vi "MOCKBEAR_Pull_Sample.vi"(0 "MOCKBEAR in":refnum<class "MOCKBEAR.lvclass">, 1 "FEA Model":refnum<class "FEA_Model.lvclass">, 5 "error in (no error)":errorcluster) -> (12 "Frequency True":dbl, 14 "Accelerometer sample":dbl[](array[numeric]), 15 "Last pin pos node":i32, 16 "Sample Time":u32, 17 "Last pin pos meter":dbl, 18 "looping":bool, 19 "error out":errorcluster)   [LabVIEW 2021, in "MOCKBEAR.lvclass"]
uses:
  MOCKBEAR.lvclass
  FEA_Model/FEA_Model.lvclass
  MOCKBEAR.lvclass/MOCKBEAR.ctl
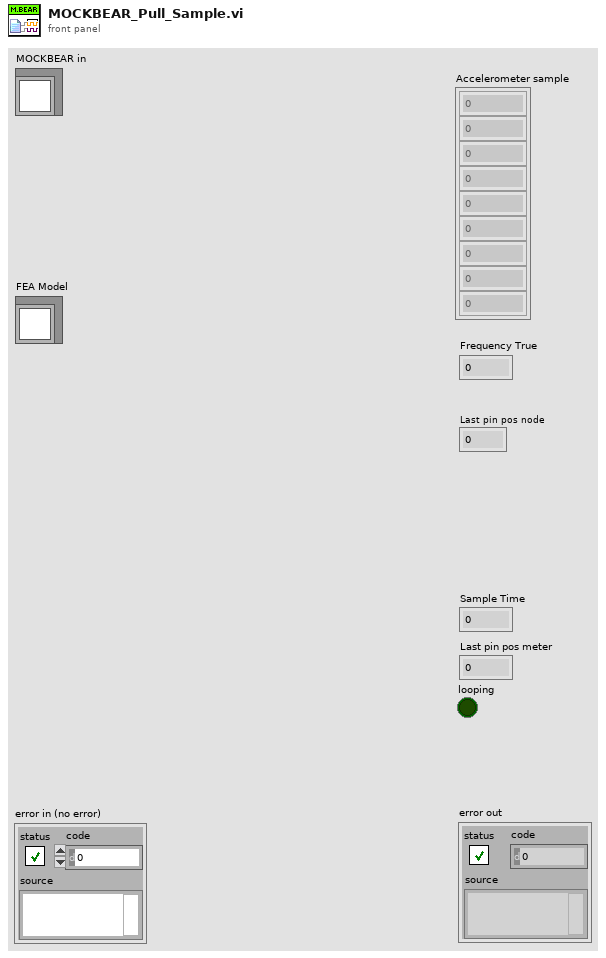
[diagram p1: front panel]
types:
  T1 = enum16{"Scalar Particle to Meter", "Scalar Node to Meter", "Scalar Meter to Particle", "Scalar Meter to Node", "Array Particle to Meter", "Array Node to Meter", "Array Meter to Particle", "Array Meter to Node"}
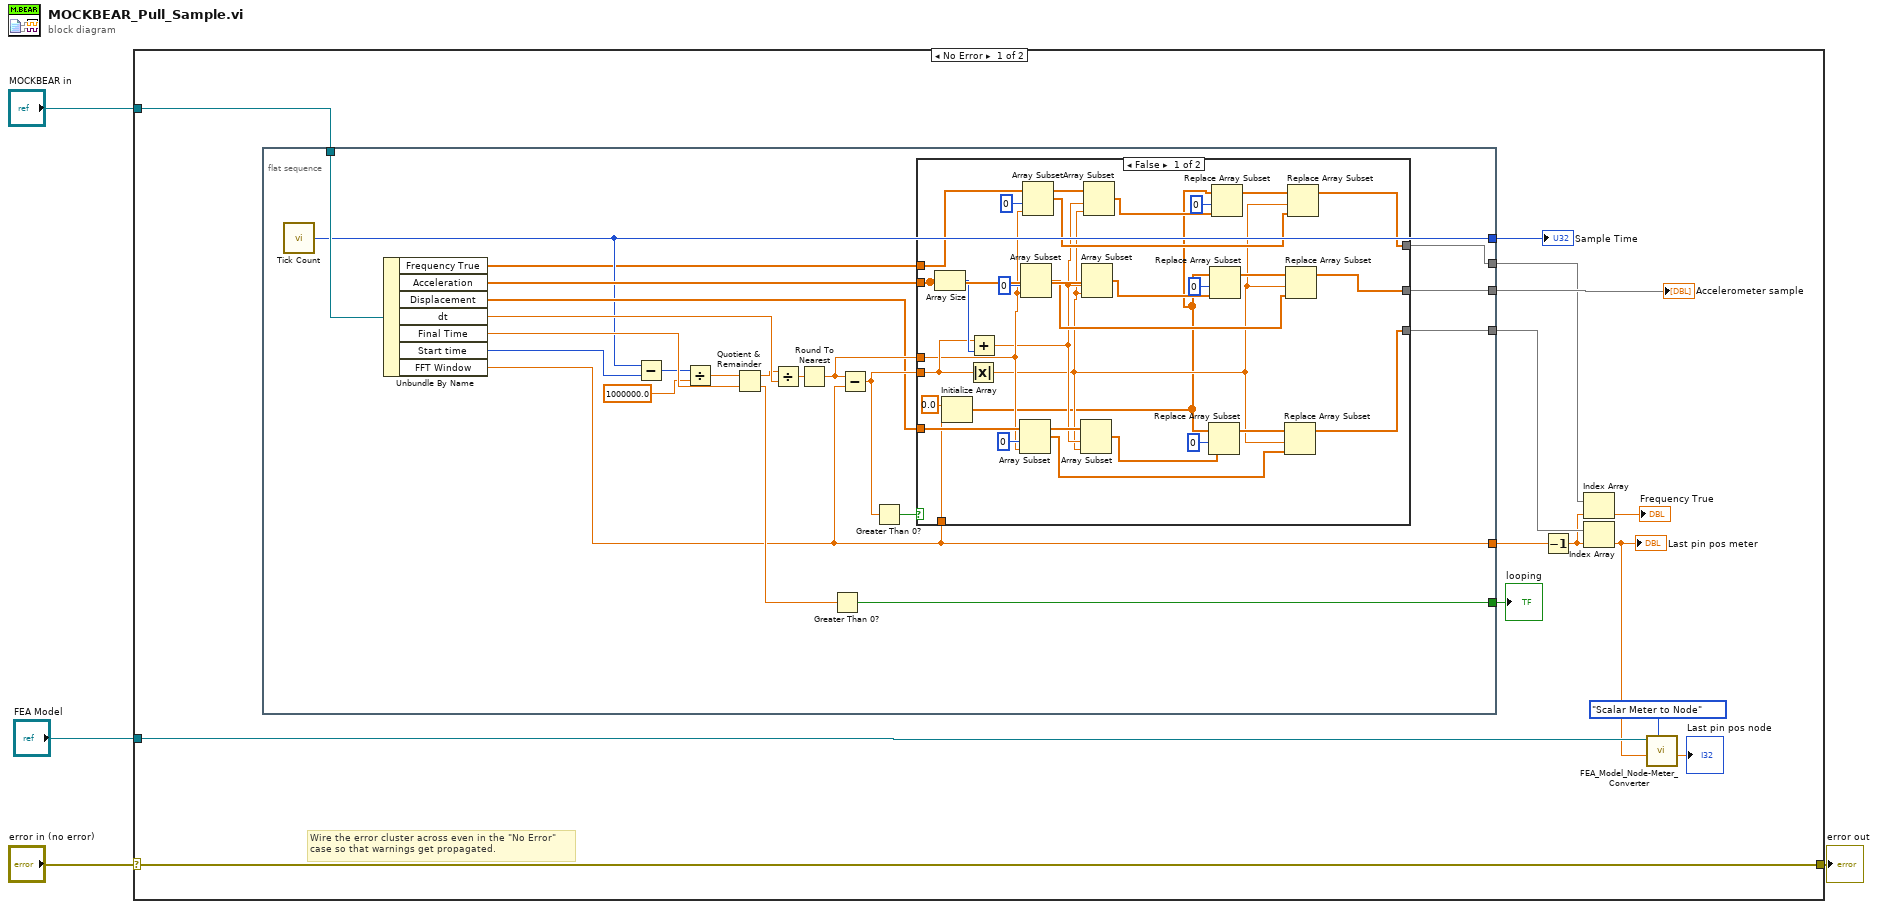
[diagram p0: block diagram]
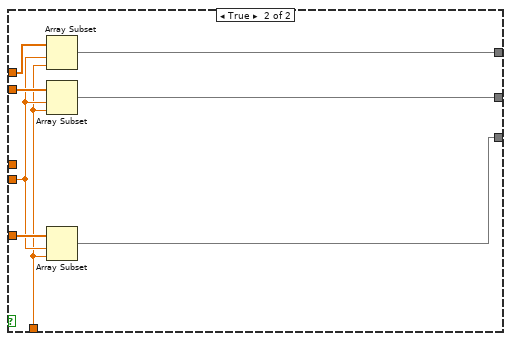
[diagram p2: hidden frame]
diagram:
  n1 = case shown="No Error" "error in (no error)" {
    selector: "error in (no error)" -> [w18 w78]
    tunnel: [w18 w78] -> w3
    tunnel: "MOCKBEAR in" -> [w9 _]
    tunnel: "FEA Model" -> [w12 _]
    frame No Error {
      # "Wire the error cluster across even in the \"No Error\"\ncase so that warnings get propagated."
      n2 = flat-sequence {
        tunnel: w9 -> [w40]
        tunnel: [w37] -> w17
        tunnel: [w33] -> w14
        tunnel: [w28] -> w16
        tunnel: [w21] -> w15
        tunnel: [w26] -> w13
        tunnel: [w19] -> w7
        frame #0 {
          n3 = call "Tick Count"() -> ("Tick Count(uSec)"=w28:u32)
          n4 = Unbundle By Name(w40) -> ("Frequency True"=w20:dbl[], "Acceleration"=w38:dbl[], "Displacement"=w30:dbl[], "dt"=w31:dbl, "Final Time"=w32:dbl, "Start time"=w29:u32, "FFT Window"=w21:dbl)
          n5 = Subtract(x=w28, y=w29) -> (x-y=w23:u32)
          n6 = Divide(x=w23, y=1000000.0) -> (x/y=w24:dbl)
          n7 = Quotient & Remainder(x=w24, y=w32) -> (x-y*floor(x/y)=w27:dbl, floor(x/y)=w25:dbl)
          n8 = Divide(x=w27, y=w31) -> (x/y=w39:dbl)
          n9 = Round To Nearest(number=w39) -> (nearest integer value=w34:dbl)
          n10 = Greater Than 0?(x=w25) -> (x > 0?=w26:bool)
          n11 = Subtract(x=w34, y=w21) -> (x-y=w35:dbl)
          n12 = Greater Than 0?(x=w35) -> (x > 0?=w36:bool)
          n13 = case shown="False" w36 {
            tunnel: w35 -> [w61 w72]
            tunnel: w38 -> [w69 w77]
            tunnel: [w64 w76] -> w37
            tunnel: w34 -> [w46 _]
            tunnel: [w60 w74] -> w33
            tunnel: w30 -> [w55 w75]
            tunnel: w21 -> [w52 w71]
            tunnel: w20 -> [w44 w73]
            tunnel: [w42 w70] -> w19
            frame False {
              n14 = Array Size(array=w69) -> (size(s)=w68:i32)
              n15 = Initialize Array(0.0 ("element"), w52) -> (w41:dbl[])
              n16 = Absolute Value(x=w61) -> (abs(x)=w43:dbl)
              n17 = Add(x=w61, y=w68) -> (x+y=w45:dbl)
              n18 = Array Subset(array=w55, index=0, length=w46) -> (w54:dbl[])
              n19 = Array Subset(array=w69, index=0, length=w46) -> (w59:dbl[])
              n20 = Array Subset(array=w44, index=0, length=w46) -> (w47:dbl[])
              n21 = Array Subset(array=w55, index=w45, length=w43) -> (w53:dbl[])
              n22 = Array Subset(array=w69, index=w45, length=w43) -> (w63:dbl[])
              n23 = Array Subset(array=w44, index=w45, length=w43) -> (w49:dbl[])
              n24 = Replace Array Subset(array=w41, new element=w53, index=0) -> (w58:dbl[])
              n25 = Replace Array Subset(array=w41, new element=w63, index=0) -> (w65:dbl[])
              n26 = Replace Array Subset(array=w41, new element=w49, index=0) -> (w50:dbl[])
              n27 = Replace Array Subset(array=w58, new element=w54, index=w43) -> (w60:dbl[])
              n28 = Replace Array Subset(array=w65, new element=w59, index=w43) -> (w64:dbl[])
              n29 = Replace Array Subset(array=w50, new element=w47, index=w43) -> (w42:dbl[])
            }
            frame True {
              n30 = Array Subset(array=w73, index=w72, length=w71) -> (w70:dbl[])
              n31 = Array Subset(array=w77, index=w72, length=w71) -> (w76:dbl[])
              n32 = Array Subset(array=w75, index=w72, length=w71) -> (w74:dbl[])
            }
          }
        }
      }
      n33 = Decrement(x=w15) -> (x-1=w5:dbl)
      n34 = Index Array(array=w7, index=w5) -> (element=→"Frequency True":dbl)
      n35 = Index Array(array=w14, index=w5) -> (element=w8:dbl)
      "Last pin pos meter" <- w8
      n36 = call "FEA_Model_Node-Meter_Converter.vi"("Conversion Mode"=T1."Scalar Meter to Node", "Scalar in"=w8, "FEA_Model in"=w12) -> ("Scalar out"=→"Last pin pos node":dbl)  [unwired: 5 in, 3 out]
      "Accelerometer sample" <- w17
      "Sample Time" <- w16
      "looping" <- w13
    }
    frame Error {
    }
  }
  "error out" <- w3
